vi "Percent to Torque Request.vi"(9 "Enabled":bool, 11 "Throttle %":dbl) -> (2 "MTorqueRequest":sgl)   [LabVIEW 2015]
uses:
  Global Data.vi
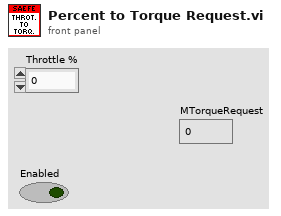
[diagram p1: front panel]
types:
  T1 = typedef "DashDriverInputs.ctl" = cluster{"ButtonsBitArray":u8, "NRedRotary":u8, "NYellowRotary":u8, "NBlackRotary":u8}
  T2 = typedef "MC Position.ctl" = cluster{"aMotor":dbl, "nMotor":dbl, "fMCOutput":dbl, "aDeltaResolverFilt":dbl}
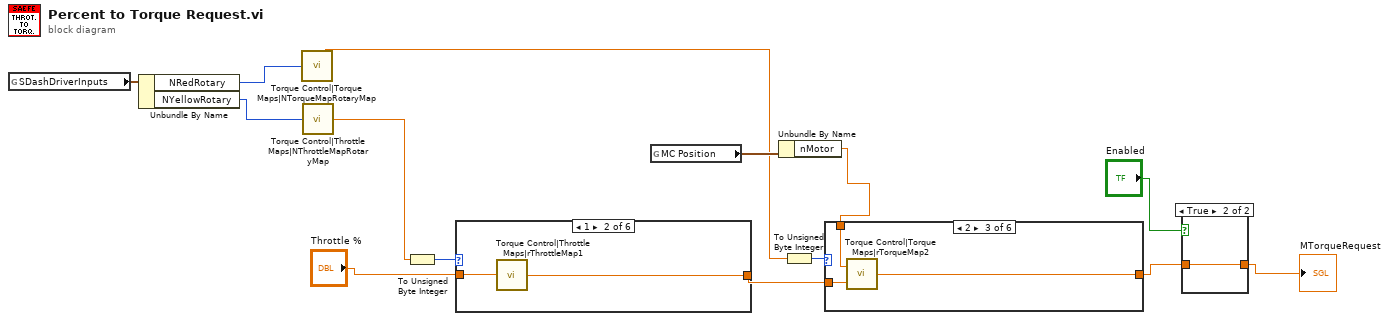
[diagram p0: block diagram]
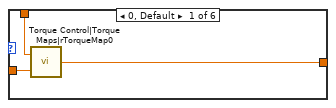
[diagram p2: hidden frame]
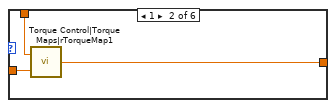
[diagram p3: hidden frame]
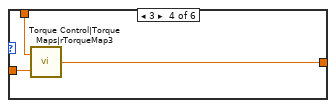
[diagram p4: hidden frame]
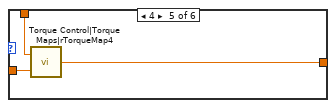
[diagram p5: hidden frame]
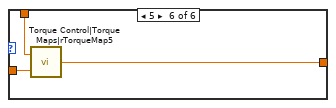
[diagram p6: hidden frame]
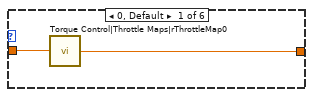
[diagram p7: hidden frame]
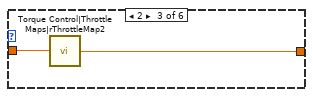
[diagram p8: hidden frame]
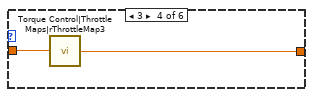
[diagram p9: hidden frame]
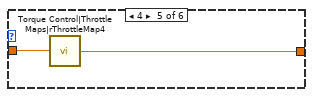
[diagram p10: hidden frame]
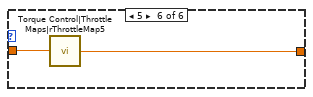
[diagram p11: hidden frame]
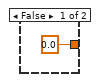
[diagram p12: hidden frame]
diagram:
  n1 = global read "Global Data.vi" "SDashDriverInputs"() -> (w11:T1)
  n2 = Unbundle By Name(w11) -> ("NRedRotary"=w3:u8, "NYellowRotary"=w1:u8)
  n3 = call "Torque Control|Torque Maps|NTorqueMapRotaryMap"("X Index"=w3) -> ("Y"=w7:sgl)
  n4 = call "Torque Control|Throttle Maps|NThrottleMapRotaryMap"("X Index"=w1) -> ("Y"=w9:sgl)
  n5 = To Unsigned Byte Integer(number=w9) -> (unsigned 8bit integer=w10:u8)
  n6 = case shown="1" w10 {
    tunnel: "Throttle %" -> [w16 w18 w20 w22 w24 w26]
    tunnel: [w15 w17 w19 w21 w23 w25] -> w12
    frame 0, Default {
      n7 = call "Torque Control|Throttle Maps|rThrottleMap0"("X Index"=w16) -> ("Y"=w15:sgl)
    }
    frame 1 {
      n8 = call "Torque Control|Throttle Maps|rThrottleMap1"("X Index"=w18) -> ("Y"=w17:sgl)
    }
    frame 2 {
      n9 = call "Torque Control|Throttle Maps|rThrottleMap2"("X Index"=w20) -> ("Y"=w19:sgl)
    }
    frame 3 {
      n10 = call "Torque Control|Throttle Maps|rThrottleMap3"("X Index"=w22) -> ("Y"=w21:sgl)
    }
    frame 4 {
      n11 = call "Torque Control|Throttle Maps|rThrottleMap4"("X Index"=w24) -> ("Y"=w23:sgl)
    }
    frame 5 {
      n12 = call "Torque Control|Throttle Maps|rThrottleMap5"("X Index"=w26) -> ("Y"=w25:sgl)
    }
  }
  n13 = global read "Global Data.vi" "MC Position"() -> (w13:T2)
  n14 = Unbundle By Name(w13) -> ("nMotor"=w2:dbl)
  n15 = To Unsigned Byte Integer(number=w7) -> (unsigned 8bit integer=w8:u8)
  n16 = case shown="2" w8 {
    tunnel: w2 -> [w29 w32 w35 w38 w41 w44]
    tunnel: w12 -> [w28 w31 w34 w37 w40 w43]
    tunnel: [w27 w30 w33 w36 w39 w42] -> w5
    frame 0, Default {
      n17 = call "Torque Control|Torque Maps|rTorqueMap0"("Y Index"=w28, "X Index"=w29) -> ("Z"=w27:sgl)
    }
    frame 1 {
      n18 = call "Torque Control|Torque Maps|rTorqueMap1"("Y Index"=w31, "X Index"=w32) -> ("Z"=w30:sgl)
    }
    frame 2 {
      n19 = call "Torque Control|Torque Maps|rTorqueMap2"("Y Index"=w34, "X Index"=w35) -> ("Z"=w33:sgl)
    }
    frame 3 {
      n20 = call "Torque Control|Torque Maps|rTorqueMap3"("Y Index"=w37, "X Index"=w38) -> ("Z"=w36:sgl)
    }
    frame 4 {
      n21 = call "Torque Control|Torque Maps|rTorqueMap4"("Y Index"=w40, "X Index"=w41) -> ("Z"=w39:sgl)
    }
    frame 5 {
      n22 = call "Torque Control|Torque Maps|rTorqueMap5"("Y Index"=w43, "X Index"=w44) -> ("Z"=w42:sgl)
    }
  }
  n23 = case shown="True" "Enabled" {
    tunnel: w5 -> [_ w46]
    tunnel: [0.0 w46] -> w4
    frame False {
    }
    frame True {
    }
  }
  "MTorqueRequest" <- w4
